vi "GetProperties.vi"(8 "error in":errorcluster, 11 "Slide in":refnum<class "Slide.lvclass">) -> (0 "error out":errorcluster, 3 "Slide out":refnum<class "Slide.lvclass">)   [LabVIEW 2014, in "Slide.lvclass"]
uses:
  Slide.lvclass
  Slide.lvclass/Slide.ctl
  NumericWithScale/NumericWithScale.lvclass
  SlideScale/SlideScale.lvclass
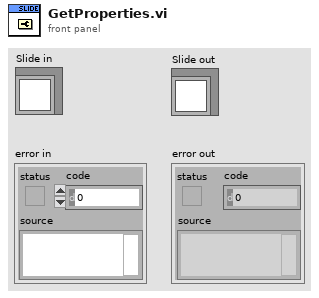
[diagram p1: front panel]
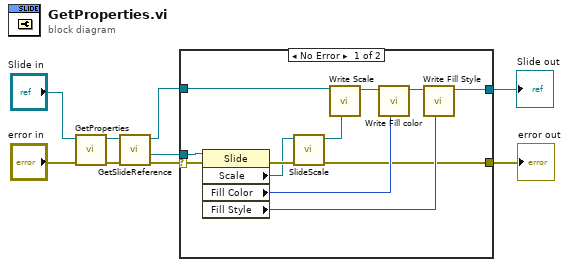
[diagram p0: block diagram]
diagram:
  n1 = call-parent "GetProperties.vi"("error in"="error in", "NumericWithScale in"="Slide in") -> ("error out"=w6:errorcluster, "NumericWithScale out"=w7:refnum<class "Slide.lvclass">)  [unwired: 8 in]
  n2 = call "GetSlideReference.vi"("error in"=w6, "Slide in"=w7) -> ("error out"=w4:errorcluster, "slide reference"=w3:refnum<vi>, "Slide out"=w5:refnum<class "Slide.lvclass">)  [unwired: 7 in]
  n3 = case shown="No Error" w4 {
    selector: w4 -> [w21 w22]
    tunnel: w5 -> [w10 w23]
    tunnel: w3 -> [w20 _]
    tunnel: [w15 w23] -> w2
    tunnel: [w13 w22] -> w1
    frame No Error {
      n4 = property class="Slide"(reference=w20, error in=w21) -> (error out=w14:errorcluster, "Scale"=w12:refnum<vi>, "Fill Color"=w19:u32, "Fill Style"=w18:i32)  [unwired: 1 out]
      n5 = call "SlideScale.vi"("error in"=w14, "Gen Refnum"=w12) -> ("error out"=w13:errorcluster, "SlideScale out"=w11:refnum<class "SlideScale.lvclass">)  [unwired: 8 in]
      n6 = call "Write Scale.vi"("Scale"=w11, "Slide in"=w10) -> ("Slide out"=w16:refnum<class "Slide.lvclass">)  [unwired: 7 in]
      n7 = call "Write Fill color.vi"("Fill color"=w19, "Slide in"=w16) -> ("Slide out"=w17:refnum<class "Slide.lvclass">)  [unwired: 7 in]
      n8 = call "Write Fill Style.vi"("Fill Style"=w18, "Slide in"=w17) -> ("Slide out"=w15:refnum<class "Slide.lvclass">)  [unwired: 7 in]
    }
    frame Error {
    }
  }
  "error out" <- w1
  "Slide out" <- w2
